vi "TIFF_2_Create_Bitmap_Metadata.vi"(8 "error in (no error)":errorcluster, 9 "Input cluster":T2, 10 "Taggs":T1={"Date/Time"="/ifd/{ushort=306}", "System model"="/ifd/{ushort=272}", "Software version"="/ifd/{ushort=305}", "Copyright"="/ifd/{ushort=33432}", "User"="/ifd/{ushort=315}", "Description"="/ifd/{ushort=270}", "X resolution"="/ifd/{ushort=282}", "Y resolution"="/ifd/{ushort=283}", "Resolution unit"="/ifd/{ushort=296}"}, 11 "Metadata IN":T1={"Date/Time"="15:07:2025 15:22:10", "System model"="Spinning Polar - 110", "Software version"="Labview - Polar_v2.0.lvproj", "Copyright"="IF - CNRS - AMU - CentraleMed - Mailfert - Honorine", "User"="Sophie Brasselet", "Description"="Embryo - GFP-Septin - RFP-Myosin", "X resolution"="125", "Y resolution"="125", "Resolution unit"="nm"}) -> (0 "Error Out":errorcluster, 1 "Output cluster":T2)   [LabVIEW 2025]
doc: "This software was created to prototype writing metadata to a TIFF file with a single image.\n\n<B>Usage:</B> This software is free to use, copy or plagiariaze. It is provided \"as-is\", and no technical support will be provided. The copyright is retained by NASA Marshall Space Flight Center.\n\n<B>Testing:</B> This software was tested by A) verifying that operations were completed successfully using LabVIEW 2009 on Windows XP, .NET version 4.0 and B) Windows Vista Microsoft Office Picture Manager was able to read and display the output file and C) Windows Vista Windows Photo Gallery was able to read and display the output file and the Description and D) Adobe Photoshop for Macintosh was able to correctly load and display the image and all the metadata.\n\n<B>Note:</B> This software requires .NET version 4.0\n\n<B>Warning:</B> This software will overwrite the destination file if it exists.\n\nThis software originally developed by:\nDerek Mayer\nBAE Systems - Technology Solutions & Services\n308 Voyager Way\nHuntsville, AL 35806\n(256) 890-8000\nwww.mevatec.com\nwww.baesystems.com/TSS\nSeptember 2010"
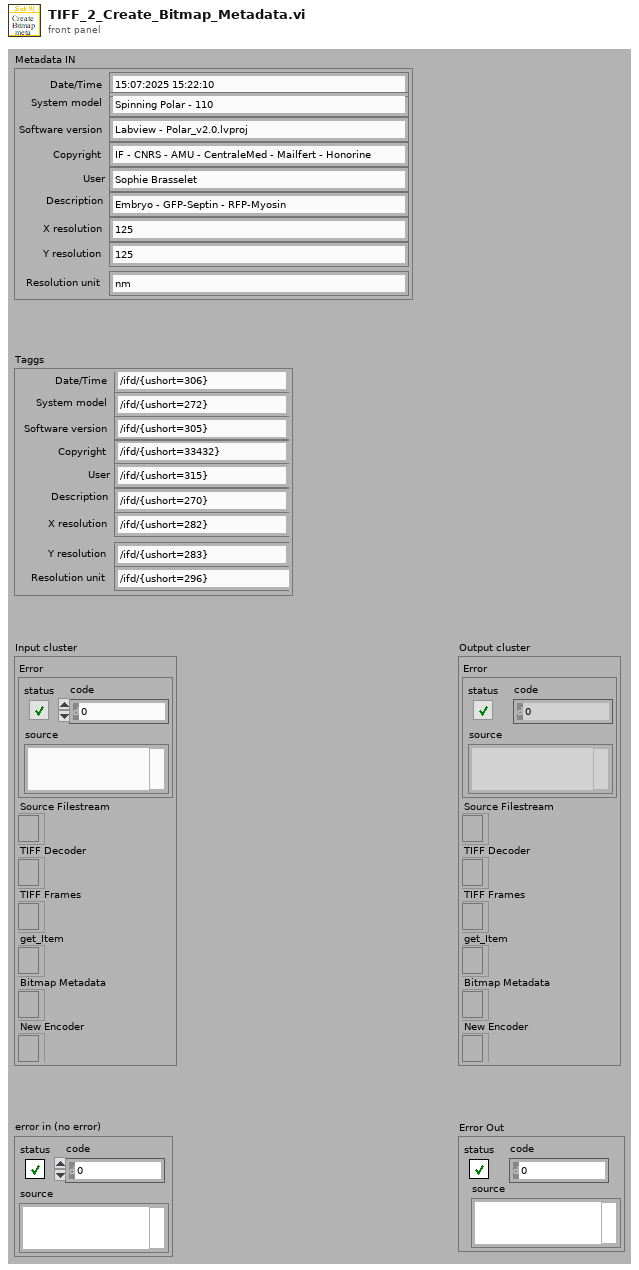
[diagram p1: front panel]
types:
  T1 = cluster{"Date/Time":string, "System model":string, "Software version":string, "Copyright":string, "User":string, "Description":string, "X resolution":string, "Y resolution":string, "Resolution unit":string}
  T2 = cluster{"Error":errorcluster, "Source Filestream":refnum<k24>, "TIFF Decoder":refnum<k24>, "TIFF Frames":refnum<k24>, "get_Item":refnum<k24>, "Bitmap Metadata":refnum<k24>, "New Encoder":refnum<k24>}
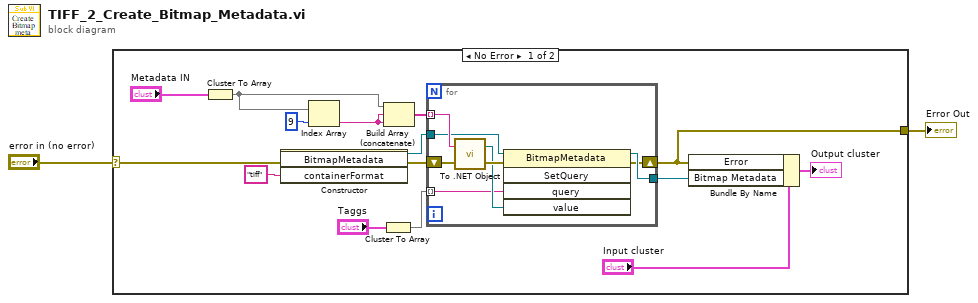
[diagram p0: block diagram]
diagram:
  n1 = case shown="No Error" "error in (no error)" {
    selector: "error in (no error)" -> [w17 w26]
    tunnel: [w5 w26] -> w1
    frame No Error {
      n2 = Cluster To Array(cluster="Metadata IN") -> (array=w14:string[])
      n3 = constructor class="BitmapMetadata"(error in=w17, "containerFormat"="tiff") -> (reference out=w11:refnum<k24>, error out=w12:errorcluster)  [unwired: 2 in, 2 out]
      n4 = Index Array(array=w14, index=9) -> (element=w13:string)
      n5 = Cluster To Array(cluster="Taggs") -> (array=w16:string[])
      n6 = Build Array (concatenate)(w14, w13, w13) -> (w15:string[])
      n7 = for {
        tunnel: [w22] -> w7
        tunnel: w11 -> [w19]
        shift-right: [w20] -> w5
        shift-left: w12 -> [w25]
        tunnel: w16 -> [w18] mode=indexing
        tunnel: w15 -> [w21] mode=indexing
        n8 = call <vilib>:"To .NET Object.vi"("error in (no error)"=w25, "anything"=w21) -> ("error out"=w24:errorcluster, ".NET object"=w23:refnum<k24>)
        n9 = invoke class="BitmapMetadata" method="SetQuery"(reference=w19, error in=w24, "query"=w18, "value"=w23) -> (reference out=w22:refnum<k24>, error out=w20:errorcluster)  [unwired: 1 in, 3 out]
      }
      n10 = Bundle By Name(cluster="Input cluster", "Error"=w5, "Bitmap Metadata"=w7) -> (→"Output cluster":T2)
    }
    frame Error {
    }
  }
  "Error Out" <- w1
